vi "controlAlejamiento.vi"(6 "z thr":dbl=250.0 format="%#_13g", 7 "controlP":T1, 8 "error in (no error)":errorcluster, 9 "stp":dbl, 10 "Y":dbl, 11 "X":dbl) -> (0 "error out":errorcluster, 3 "Z":dbl)   [LabVIEW 2018]
uses:
  <vilib>/Analysis/NI_AALPro.lvlib
panel:
  out "VaiInc":dbl
  out "Amplitud Multimetro":dbl[](graph)
  out "Der 3":dbl[](graph)
  out "Der":dbl[](graph)
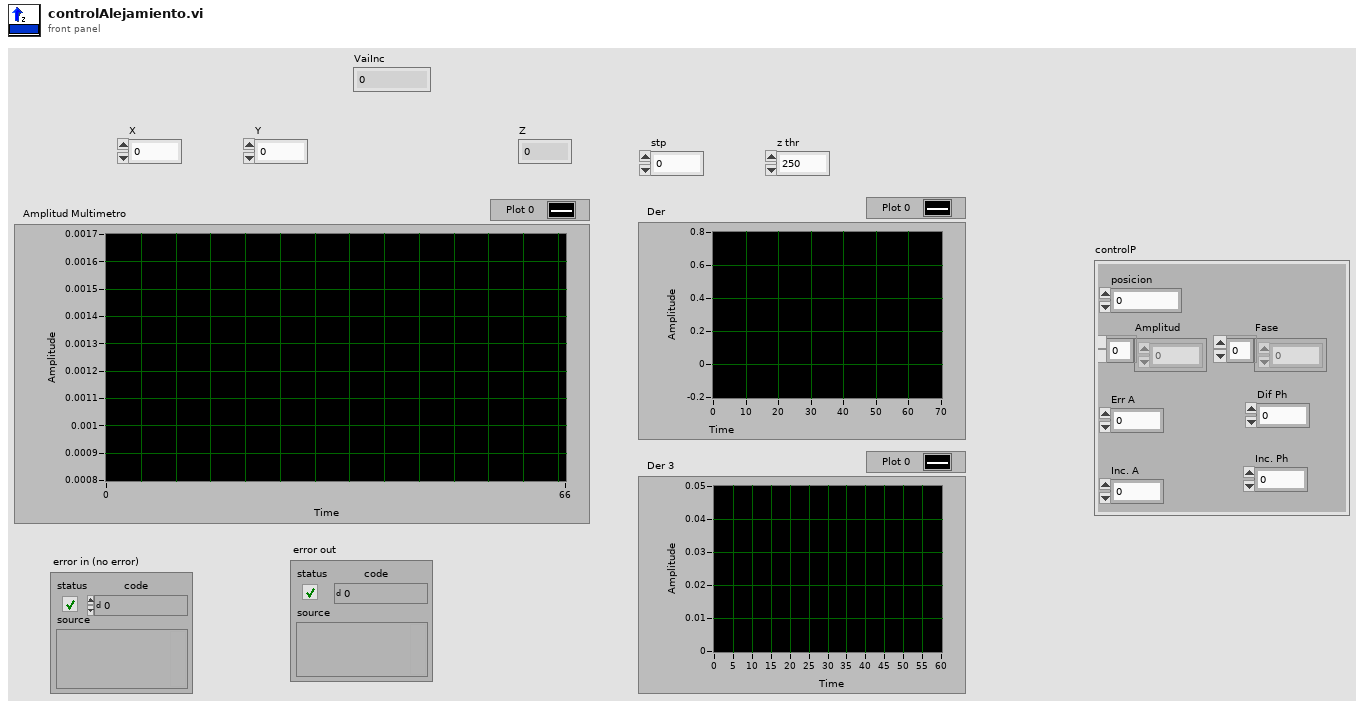
[diagram p1: front panel]
types:
  T1 = cluster{"posicion":dbl, "Amplitud":dbl[], "Fase":dbl[], "Err A":dbl, "Dif Ph":dbl, "Inc. A":dbl, "Inc. Ph":dbl}
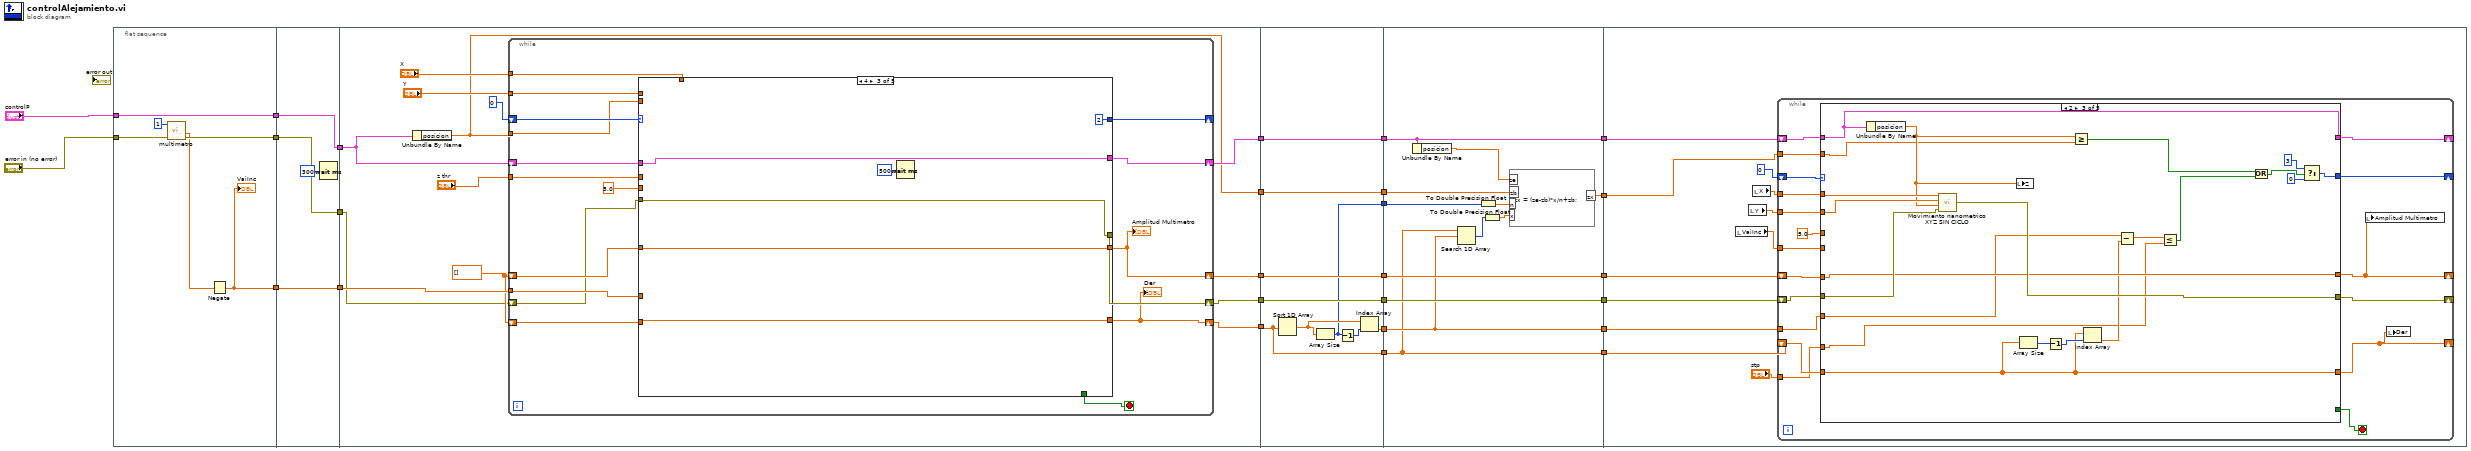
[diagram p0: block diagram]
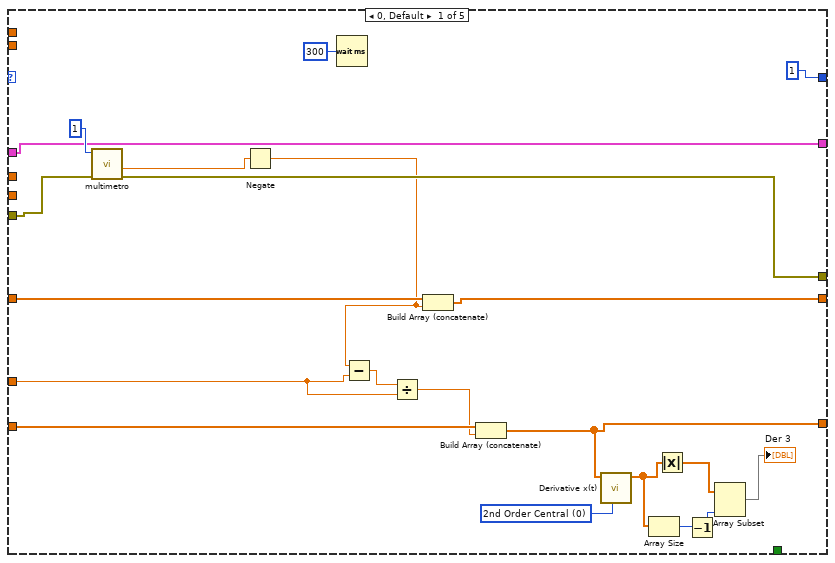
[diagram p2: hidden frame]
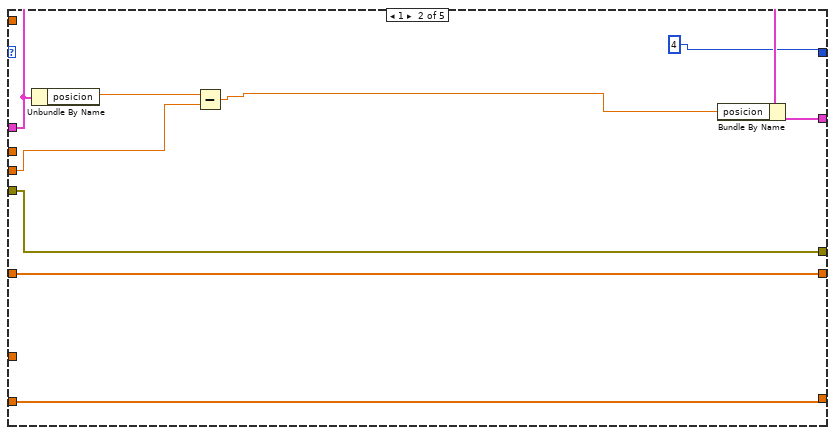
[diagram p3: hidden frame]
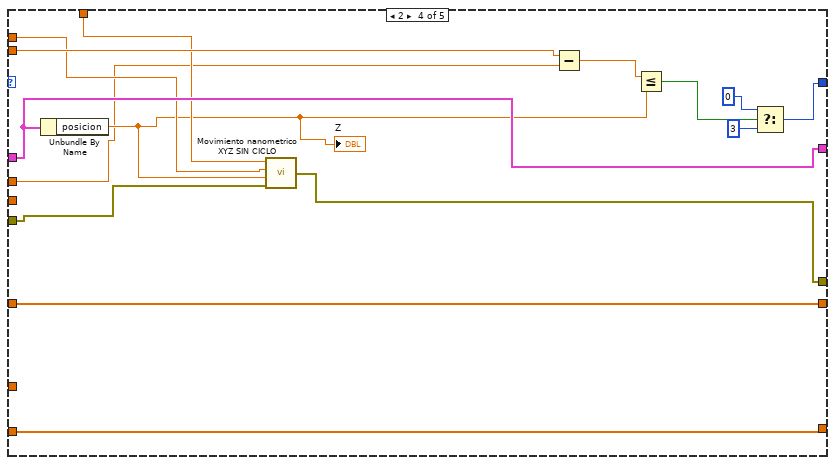
[diagram p4: hidden frame]
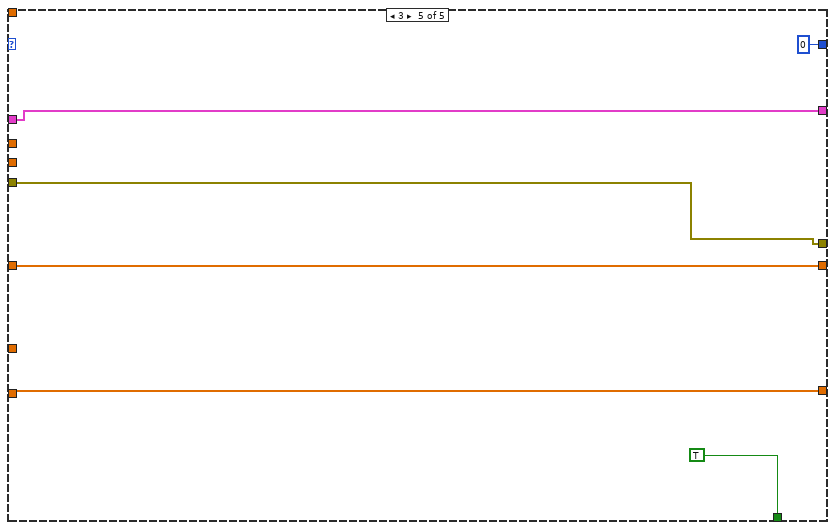
[diagram p5: hidden frame]
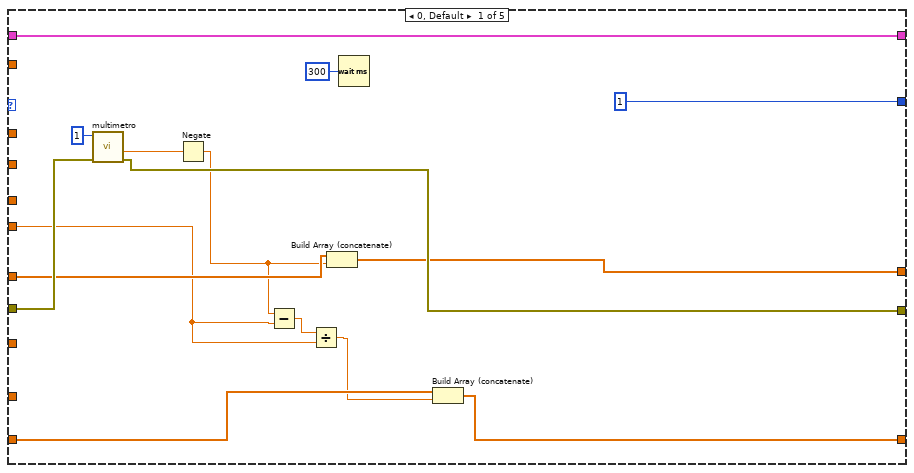
[diagram p6: hidden frame]
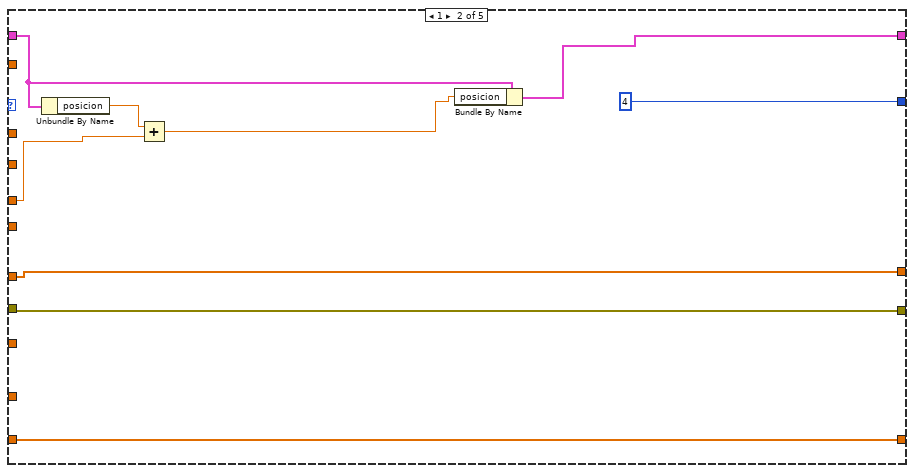
[diagram p7: hidden frame]
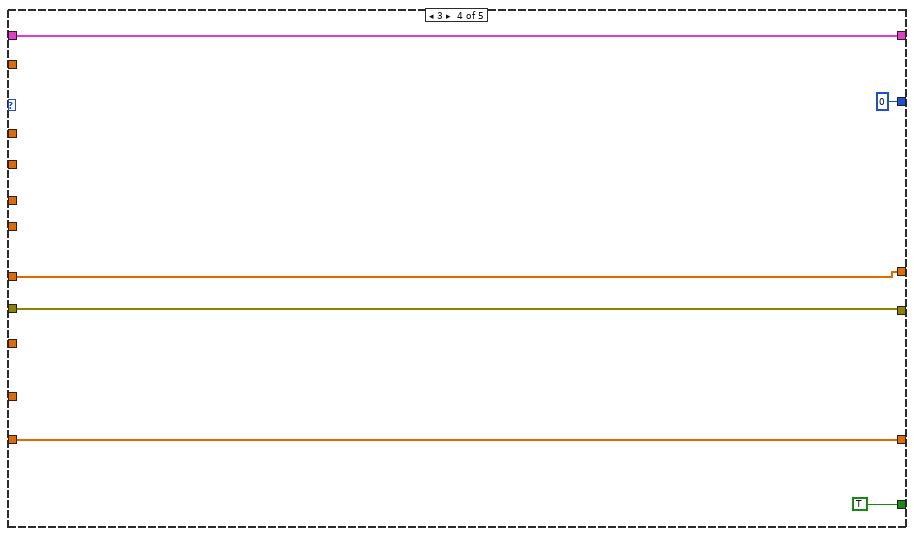
[diagram p8: hidden frame]
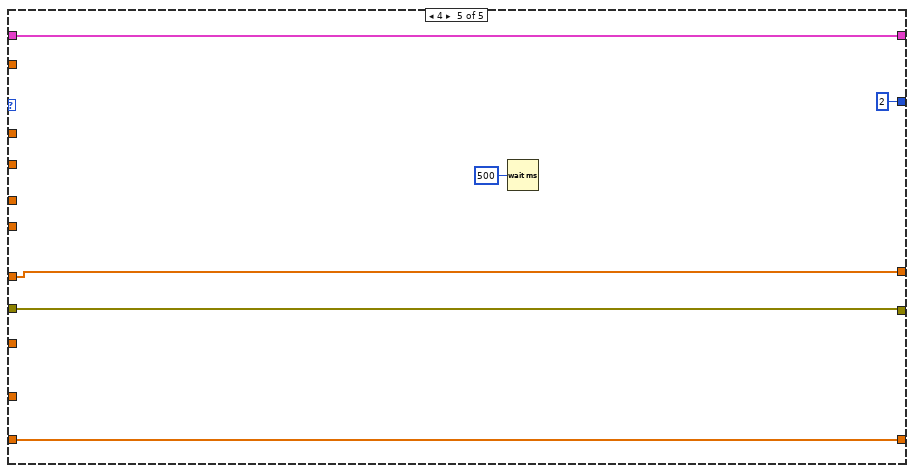
[diagram p9: hidden frame]
diagram:
  n1 = flat-sequence {
    tunnel: "error in (no error)" -> [w31]
    tunnel: [w30] -> w24
    tunnel: [w27] -> w22
    tunnel: [w29] -> w20
    tunnel: "controlP" -> [w29]
    tunnel: [w35] -> w25
    tunnel: w24 -> [w35]
    tunnel: [w34] -> w23
    tunnel: w22 -> [w34]
    tunnel: [w33] -> w21
    tunnel: w20 -> [w33]
    tunnel: w25 -> [w40]
    tunnel: w23 -> [w49]
    tunnel: w21 -> [w47]
    tunnel: [w42] -> w18
    tunnel: [w41] -> w17
    tunnel: [w39] -> w16
    tunnel: [w38] -> w15
    tunnel: [w37] -> w1
    tunnel: w18 -> [w129]
    tunnel: [w130] -> w14
    tunnel: [w129] -> w12
    tunnel: [w128] -> w10
    tunnel: w17 -> [w128]
    tunnel: [w127] -> w8
    tunnel: w16 -> [w127]
    tunnel: [w126] -> w6
    tunnel: w15 -> [w126]
    tunnel: [w125] -> w3
    tunnel: [w124] -> w2
    tunnel: w1 -> [w124]
    tunnel: w14 -> [w134]
    tunnel: [w134] -> w13
    tunnel: w12 -> [w133]
    tunnel: [w133] -> w11
    tunnel: w10 -> [w135]
    tunnel: [w135] -> w9
    tunnel: w8 -> [w144]
    tunnel: [w144] -> w7
    tunnel: w6 -> [w140]
    tunnel: [w140] -> w5
    tunnel: [w143] -> w4
    tunnel: w3 -> [w141]
    tunnel: w2 -> [w138]
    tunnel: w13 -> [w155]
    tunnel: w11 -> [w153]
    tunnel: w9 -> [w152]
    tunnel: w7 -> [w151]
    tunnel: w5 -> [w150]
    tunnel: w4 -> [w145]
    frame #0 {
      n2 = call "multimetro.vi"("error in (no error)"=w31, "mediciones"=1) -> ("error out"=w30:errorcluster, "voltajeProm"=w28:dbl)  [unwired: 7 in, 1 out]
      n3 = Negate(x=w28) -> (-x=w27:dbl)
      "VaiInc" <- w27
    }
    frame #1 {
      n4 = Wait (ms)(milliseconds to wait=u32 300) -> ()  [unwired: 1 out]
    }
    frame #2 {
      w46 = dbl[] []
      n5 = Unbundle By Name(w47) -> ("posicion"=w37:dbl)
      n6 = while {
        shift-right: [w64] -> _
        shift-left: 0 -> [w66]
        shift-right: [w52] -> w41
        shift-left: w46 -> [w65]
        shift-right: [w62] -> w38
        shift-left: w47 -> [w61]
        tunnel: w37 -> [w60]
        shift-right: [w56] -> w42
        shift-left: w46 -> [w57]
        tunnel: w49 -> [w55]
        tunnel: "X" -> [w54]
        tunnel: "Y" -> [w53]
        tunnel: "z thr" -> [w51]
        shift-right: [w63] -> w39
        shift-left: w40 -> [w50]
        stop <- w58 stop-if-true
        n7 = case shown="4" w66 {
          tunnel: w65 -> [w83 w92 w98 w109 w121]
          tunnel: w50 -> [w86 w91 w99 w112 w120]
          tunnel: [1 4 2 ("f") w114 0 ("f")] -> w64
          tunnel: [w84 w91 w99 w111 w120] -> w63
          tunnel: [w82 w92 w98 w109 w121] -> w52
          tunnel: [w81 w94 w101 w110 w119] -> w62
          tunnel: w61 -> [w81 w93 w101 w110 w119]
          tunnel: w60 -> [_ _ _ w113 _]
          tunnel: 5.0 -> [_ w95 _ _ _]
          tunnel: [_ _ _ _ TRUE] -> w58
          tunnel: w57 -> [w78 w88 w97 w108 w118]
          tunnel: [w73 w88 w97 w108 w118] -> w56
          tunnel: w55 -> [w74 _ _ _ _]
          tunnel: w54 -> [_ _ _ w106 _]
          tunnel: w53 -> [_ _ _ w105 _]
          tunnel: w51 -> [_ _ _ w103 _]
          frame 0, Default {
            w72 = u16 0 items=["2nd Order Central", "4th Order Central", "Forward", "Backward"] ("method")
            n8 = call "multimetro.vi"("error in (no error)"=w86, "mediciones"=1) -> ("error out"=w84:errorcluster, "voltajeProm"=w79:dbl)  [unwired: 7 in, 1 out]
            n9 = Negate(x=w79) -> (-x=w77:dbl)
            n10 = Wait (ms)(milliseconds to wait=u32 300) -> ()  [unwired: 1 out]
            n11 = Subtract(x=w77, y=w74) -> (x-y=w76:dbl)
            n12 = Divide(x=w76, y=w74) -> (x/y=w75:dbl)
            n13 = Build Array (concatenate)(w83, w77) -> (w82:dbl[])
            n14 = Build Array (concatenate)(w78, w75) -> (w73:dbl[])
            n15 = call <vilib>:"Derivative x(t).vi"("method"=w72, "X"=w73) -> ("dX/dt"=w68:dbl[])  [unwired: 8 in, 1 out]
            n16 = Array Size(array=w68) -> (size(s)=w71:i32)
            n17 = Absolute Value(x=w68) -> (abs(x)=w67:dbl[])
            n18 = Decrement(x=w71) -> (x-1=w70:i32)
            n19 = Array Subset(array=w67, length=w70) -> (→"Der 3":dbl[])  [unwired: 1 in]
          }
          frame 1 {
            n20 = Unbundle By Name(w93) -> ("posicion"=w96:dbl)
            n21 = Subtract(x=w96, y=w95) -> (x-y=w89:dbl)
            n22 = Bundle By Name(cluster=w93, "posicion"=w89) -> (w94:T1)
          }
          frame 4 {
            n23 = Wait (ms)(milliseconds to wait=u32 500) -> ()  [unwired: 1 out]
          }
          frame 2 {
            n24 = Unbundle By Name(w110) -> ("posicion"=w104:dbl)
            "Z" <- w104
            n25 = call "Movimiento nanometrico XYZ SIN CICLO.vi"("Error In"=w112, "Movimiento en Z"=w104, "Movimiento en Y"=w105, "Movimiento en X"=w106) -> ("Error Out"=w111:errorcluster)  [unwired: 2 in]
            n26 = Subtract(x=w113, y=w103) -> (x-y=w117:dbl)
            n27 = Less Or Equal?(x=w117, y=w104) -> (x <= y?=w107:bool)
            n28 = Select(t=0, s=w107, f=3) -> (s? t:f=w114:i32)
          }
          frame 3 {
          }
        }
        "Der" <- w56
        "Amplitud Multimetro" <- w52
      }
    }
    frame #3 {
      n29 = Sort 1D Array(array=w129) -> (sorted array=w131:dbl[])
      n30 = Array Size(array=w131) -> (size(s)=w125:i32)
      n31 = Decrement(x=w125) -> (x-1=w132:i32)
      n32 = Index Array(array=w131, index=w132) -> (element=w130:dbl)
    }
    frame #4 {
      n33 = Unbundle By Name(w140) -> ("posicion"=w139:dbl)
      n34 = Search 1D Array(1D array=w133, element=w134) -> (index of element=w136:i32)  [unwired: 1 in]
      n35 = To Double Precision Float(number=w141) -> (double precision float=w142:dbl)
      n36 = To Double Precision Float(number=w136) -> (double precision float=w137:dbl)
      n37 = formula code="zx = (ze-zb)*x/n+zb;"("ze"=w139, "zb"=w138, "n"=w142, "x"=w137) -> ("zx"=w143:dbl)
    }
    frame #5 {
      n38 = local read "VaiInc"() -> (w149:dbl)
      n39 = local read "Y"() -> (w147:dbl)
      n40 = local read "X"() -> (w148:dbl)
      n41 = while {
        tunnel: w155 -> [w156]
        shift-right: [w167] -> _
        shift-left: 0 -> [w173]
        shift-right: [w157] -> _
        shift-left: w153 -> [w168]
        shift-right: [w158] -> _
        shift-left: w152 -> [w169]
        shift-right: [w170] -> _
        shift-left: w151 -> [w172]
        shift-right: [w165] -> _
        shift-left: w150 -> [w171]
        tunnel: w149 -> [w166]
        tunnel: w148 -> [w163]
        tunnel: w147 -> [w162]
        tunnel: "stp" -> [w161]
        tunnel: w145 -> [w160]
        stop <- w159 stop-if-true
        n42 = case shown="2" w173 {
          tunnel: w172 -> [w187 w191 w216 w220 w227]
          tunnel: w171 -> [w174 w195 w213 w223 w230]
          tunnel: [w185 w191 w215 w220 w227] -> w170
          tunnel: w169 -> [w184 w192 w214 w221 w228]
          tunnel: [w183 w192 w214 w221 w228] -> w158
          tunnel: [w176 w190 w210 w219 w226] -> w157
          tunnel: w168 -> [w177 w190 w210 w219 w226]
          tunnel: [1 4 w200 0 ("f") 2 ("f")] -> w167
          tunnel: w166 -> [w178 _ _ _ _]
          tunnel: [w174 w193 w213 w223 w230] -> w165
          tunnel: 5.0 -> [_ w196 _ _ _]
          tunnel: w163 -> [_ _ w218 _ _]
          tunnel: w162 -> [_ _ w217 _ _]
          tunnel: w161 -> [_ _ w207 _ _]
          tunnel: w160 -> [_ _ w205 _ _]
          tunnel: [_ _ _ TRUE _] -> w159
          tunnel: w156 -> [_ _ w198 _ _]
          frame 0, Default {
            n43 = call "multimetro.vi"("error in (no error)"=w187, "mediciones"=1) -> ("error out"=w185:errorcluster, "voltajeProm"=w186:dbl)  [unwired: 7 in, 1 out]
            n44 = Negate(x=w186) -> (-x=w180:dbl)
            n45 = Subtract(x=w180, y=w178) -> (x-y=w179:dbl)
            n46 = Divide(x=w179, y=w178) -> (x/y=w175:dbl)
            n47 = Build Array (concatenate)(w184, w180) -> (w183:dbl[])
            n48 = Wait (ms)(milliseconds to wait=u32 300) -> ()  [unwired: 1 out]
            n49 = Build Array (concatenate)(w177, w175) -> (w176:dbl[])
          }
          frame 1 {
            n50 = Unbundle By Name(w195) -> ("posicion"=w197:dbl)
            n51 = Add(x=w197, y=w196) -> (x+y=w194:dbl)
            n52 = Bundle By Name(cluster=w195, "posicion"=w194) -> (w193:T1)
          }
          frame 2 {
            n53 = Unbundle By Name(w213) -> ("posicion"=w206:dbl)
            n54 = call "Movimiento nanometrico XYZ SIN CICLO.vi"("Error In"=w216, "Movimiento en Z"=w206, "Movimiento en Y"=w217, "Movimiento en X"=w218) -> ("Error Out"=w215:errorcluster)  [unwired: 2 in]
            n55 = local write "Z"(w206) -> ()
            n56 = Array Size(array=w210) -> (size(s)=w212:i32)
            n57 = Decrement(x=w212) -> (x-1=w211:i32)
            n58 = Greater Or Equal?(x=w206, y=w205) -> (x >= y?=w204:bool)
            n59 = Index Array(array=w210, index=w211) -> (element=w209:dbl)
            n60 = Subtract(x=w198, y=w209) -> (x-y=w208:dbl)
            n61 = Less Or Equal?(x=w208, y=w207) -> (x <= y?=w203:bool)
            n62 = Or(x=w204, y=w203) -> (x .or. y?=w199:bool)
            n63 = Select(t=3, s=w199, f=0) -> (s? t:f=w200:i32)
          }
          frame 3 {
          }
          frame 4 {
            n64 = Wait (ms)(milliseconds to wait=u32 500) -> ()  [unwired: 1 out]
          }
        }
        n65 = local write "Amplitud Multimetro"(w158) -> ()
        n66 = local write "Der"(w157) -> ()
      }
    }
  }
